vi "CP Insertion.vi"(11 "Input":cdb[](array[numeric])) -> (3 "Output with CP":cdb[](array[numeric]))   [LabVIEW 2022 SP3]
doc: "Creates cyclic prefix by copying last 64 symbols and appending them to beginning frame."
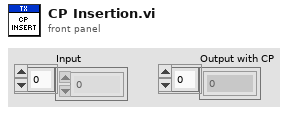
[diagram p1: front panel]
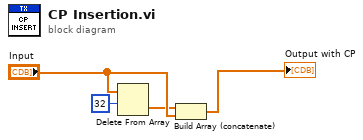
[diagram p0: block diagram]
diagram:
  n1 = Delete From Array(array="Input", length=32) -> (deleted portion=w2:cdb[])  [unwired: 1 in, 1 out]
  n2 = Build Array (concatenate)(w2, "Input") -> (→"Output with CP":cdb[])
